vi "working controller not circlre.vi"() -> ()   [LabVIEW 2017]
uses:
  <vilib>/Simulation/Scripting/Companion Diagram/SimConfigNode/SimParams.ctl
  <vilib>/Simulation/Scripting/Companion Diagram/SimConfigNode/_simSolvers.ctl
  <vilib>/Simulation/Implementation/Shared/SIMSCR Execution Mode.ctl
  <vilib>/Simulation/Param Hierarchy/Typedefs/SIMPH Param Control Actions.ctl
  <vilib>/Simulation/Implementation/Shared/NILVSim_ParamChanged.vi
  <vilib>/Simulation/Implementation/Shared/NILVSIM_BeginStep.vi
  <vilib>/Simulation/Implementation/Shared/NILVSim_Manager.vi
  <vilib>/Utility/error.llb/Clear Errors.vi
  <vilib>/Simulation/Implementation/Shared/NILVSim_FinalizeModel.vi
  <vilib>/DAQmx/read.llb/DAQmx Read (Counter DBL 1Chan 1Samp).vi
  <vilib>/DAQmx/read.llb/DAQmx Read (Digital Bool 1Line 1Point).vi
  917b7e52-755f-4d44-bea8-9e7c9beac24e.vi
  a58f9967-76f1-4ebc-ad3d-26e75a3ca160.vi
  <vilib>/DAQmx/write.llb/DAQmx Write (Analog DBL 1Chan 1Samp).vi
  <vilib>/DAQmx/create/channels.llb/DAQmx Create Channel (AO-Voltage-Basic).vi
  <vilib>/DAQmx/create/channels.llb/DAQmx Create Channel (DI-Digital Input).vi
  <vilib>/DAQmx/create/channels.llb/DAQmx Create Channel (CI-Count Edges).vi
  <vilib>/Simulation/Implementation/Shared/SIM Unbundle Sim Info.vi
  <vilib>/Simulation/Implementation/Shared/NILVSim_Initialize.vi
  <vilib>/Simulation/Utility/Implementation/NILVSim Get Time and IsAcceptedStep.vi
  <vilib>/Simulation/Implementation/Shared/SIMSH Read Queue.vi
  <vilib>/Simulation/Implementation/Shared/NILVSim_GetModelError.vi
  <vilib>/Simulation/Implementation/Shared/SIM Bundle Sim Info.vi
  <vilib>/DAQmx/miscellaneous.llb/DAQmx Fill In Error Info.vi
  <vilib>/Simulation/Implementation/XNodeFramework/SimXNode/SimX.xnode
  <vilib>/Simulation/Model Libraries/PID/SIM PID (Parallel).vi
  <vilib>/Simulation/Model Libraries/PID/SIM PID.vi
  <vilib>/Simulation/Scripting/Companion Diagram/SimConfigNode/SimDog.xnode
  <vilib>/Simulation/Model Libraries/PID/SIM PID (Academic).vi
  <vilib>/Simulation/Implementation/Shared/NI_SIM_Implementation.lvlib
panel:
  out "down":bool
  out "right":bool
  out "x entered":dbl
  out "y enetred":dbl
  out "Numeric 2":i32
  out "greater -1 x":bool
  out "less 1 x":bool
  out "d":bool
  out "c":bool
  out "b":bool
  out "direction selected":dbl
  out "circle reset":bool
  in  "part circle":T1(ring)=enum."a"
  in  "Raduis":dbl
  out "at 2f":bool
  out "Step 2J":bool
  out "Step 2H":bool
  out "Shape drawing steps":enum16{"corner", "1st switch", "reverse"}(ring)
  out "Step 2D":bool
  out "Step 2C":bool
  out "c":bool
  in  "height":dbl
  in  "length":dbl
  in  "part":T2(ring)=enum."a"
  out "Step 2A":bool
  out "Step 2B":bool
  in  "Has encoders been reset?":enum16{"don't reset", "reset"}(ring)
  out "x distance currently being travelled":dbl
  out "y distance currently being travelled":dbl
  out "error calced":dbl
  out "p1 dis 2":dbl
  out "p1 dis":dbl
  out "error y":dbl
  out "calc distance y":dbl
  out "calc distanc x":dbl
  out "error x":dbl
  out "reached y":bool
  out "reached x":bool
  out "Numeric":dbl
  in  "Draw rectangle":bool
  in  "Draw circle":bool
  out "In drawing mode":bool
  in  "Right-Down":bool
  in  "Left-Up":bool
  in  "Left-Down":bool
  in  "Right-Up":bool
  in  "right":bool
  in  "left":bool
  in  "motor 2":dbl(slide)=1.5 scale=-10.0..10.0
  in  "down":bool
  in  "up":bool
  in  "Y Length":dbl=30.0
  in  "X Length":dbl=30.0
  in  "Motor 2 encoder":tag="Dev1/ctr1"
  out "Pulses M2":dbl format="%.2f"
  in  "Motor 1 encoder":tag="Dev1/ctr0"
  out "Pulses M1":dbl format="%.2f"
  out "Right":bool
  out "Bottom":bool
  out "Left":bool
  out "Top":bool
  in  "Switch 4/Line 3":tag="Dev1/port0/line3"
  in  "Switch 3/Line 2":tag="Dev1/port0/line2"
  in  "Switch 2/Line 1":tag="Dev1/port0/line1"
  in  "Switch 1/Line 0":tag="Dev1/port0/line0"
  in  "Motor stop":bool
  in  "Motor 1":tag="Dev1/ao0"
  in  "max Voltage":dbl=10.0
  in  "Min Voltage":dbl=-10.0
  in  "Motor 2":tag="Dev1/ao1"
  in  "motor 1":dbl(slide)=1.5 scale=-10.0..10.0
  in  "stop":bool
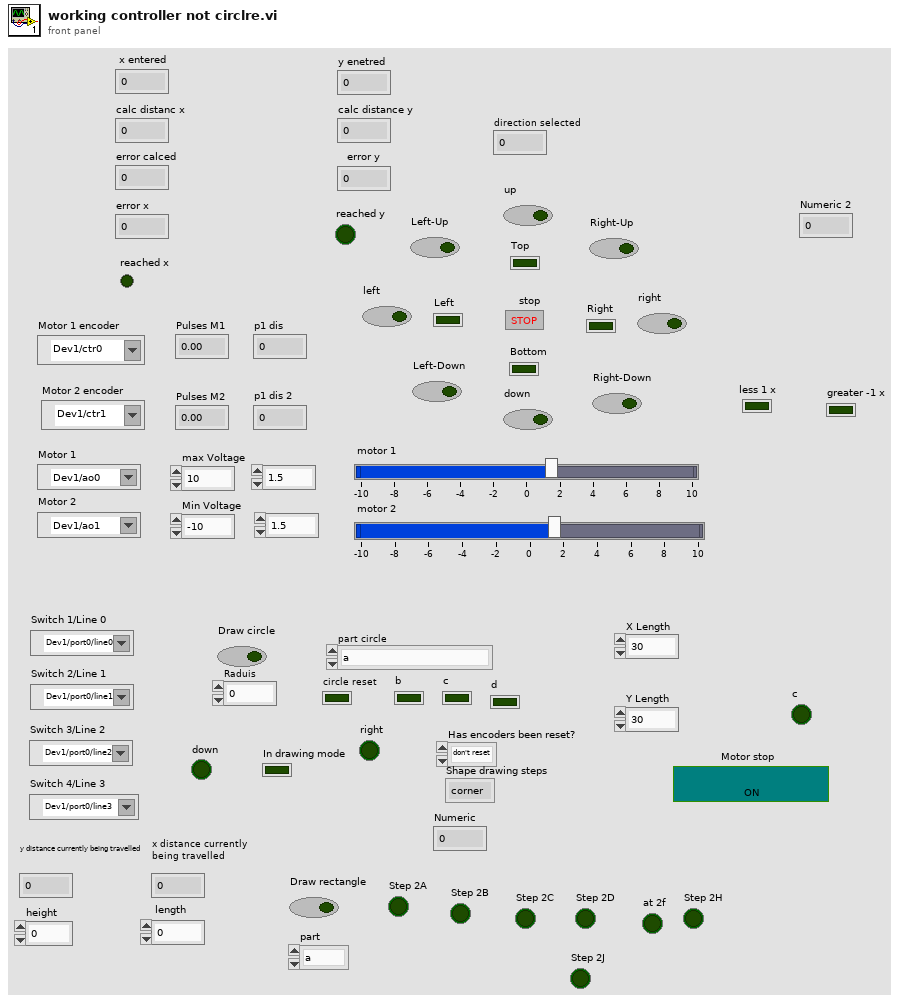
[diagram p1: front panel]
types:
  T1 = enum16{"d", "c", "b", "going right", "going down", "a"}
  T2 = enum16{"nothing", "j", "i", "h", "g", "f", "e", "d", "c", "b", "a"}
  T3 = enum16{"Simulate to Completion", "Single Time-Step Simulation (Fixed Step Only)"}
  T4 = typedef "SIMSCR Execution Mode.ctl" = enum16{"Simulate to Completion", "Single Time-Step Simulation (Fixed Step Only)"}
  T5 = typedef "SIMPH Param Control Actions.ctl" = enum16{"get params", "set params"}
  T6 = cluster{"SIMSH Sim Time":dbl, "SIM PID Derivative Gain.vi":cluster{"output":dbl}, "SIM PID Derivative Gain.vi - SIMSH":cluster{"SIMSH Sim Time":dbl, "t 3":dbl, "Select 2":cluster{"s? t:f":dbl}, "Equal?":cluster{"x = y?":bool}, "Or":cluster{"x .or. y?":bool}, "Equal To 0?":cluster{"x = 0?":bool}}, "High Frequency [s] (Tf)":dbl, "Gain":cluster{"output":dbl}, "Summation":cluster{"Result":dbl}, "Integral Gain - series.vi":cluster{"output":dbl}, "Integral Gain - series.vi - SIMSH":cluster{"SIMSH Sim Time":dbl, "Select 2":cluster{"s? t:f":dbl}, "integral in gain?":bool, "Integrator":cluster{"output y(t)":dbl}, "Gain 2":cluster{"output":dbl}, "Select":cluster{"s? t:f":dbl}, "Equal To 0?":cluster{"x = 0?":bool}, "Reciprocal":cluster{"1/x":dbl}}}
  T7 = typedef "SimParams.ctl" = cluster{"Initial Time (s)":dbl, "Final Time (s)":dbl, "Step Size (s)":dbl, "ODE Solver":T8, "Minimum Step Size (s)":dbl, "Maximum Step Size (s)":dbl, "Relative Tolerance":dbl, "Absolute Tolerance":dbl, "Software Timing":bool, "Initial Step Size (s)":dbl, "Automatic Fixed Step Size?":bool, "Automatic Discrete Step Size?":bool, "Discrete Step Size (s)":dbl, "Calculate using Time Step":bool, "Solver Wired?":bool, "Prev.Frm.Expected End":u64, "Prev.Frm.Actual End":u64, "Prev.Frm.Finished Late?":bool, "Prev.Iter.Expected End":u64, "Prev.Iter.Actual End":u64, "Prev.Iter.Finished Late?":bool, "Expected Iteration Start":u64, "Actual Iteration Start":u64, "Expected Frame Start":u64, "Actual Frame Start":u64, "Source Name":string, "Name":string, "Period":i64, "Deadline":i64, "Offset":i64, "Start":i64, "Priority":i32, "Timeout":i32, "Processor":i32, "Mode":enum32{"No Change", "Process missed periods, maintain original phase", "Discard missed periods, maintain original phase", "Process missed periods, ignore original phase", "Discard missed periods, ignore original phase"}, "Wakeup reason":enum32{"Normal", "Aborted", "Asynchronous wakeup", "Timing source error", "Timed loop error", "Timeout"}, "Error":errorcluster, "Source Type":string, "Secondary Source Type":string, "Global End Time":u64, "Global Start Time":u64, "Full Solver Reset":bool, "Execution Mode":T4, "Nan/Inf Check":bool, "Custom Solver Library":string, "Solver Is Variable":bool, "custom solver name":string, "Signal Collection Decimation":u32}
  T8 = typedef "_simSolvers.ctl" = enum16{"Runge-Kutta 1 (Euler)", "Runge-Kutta 2", "Runge-Kutta 3", "Runge-Kutta 4", "Runge-Kutta 23 (variable)", "Runge-Kutta 45 (variable)", "BDF (variable)", "Adams-Moulton (variable)", "Rosenbrock (variable)", "Discrete States Only", "SDIRK 4 (variable)", "Radau 5 (variable)", "Radau 9 (variable)", "Radau 13 (variable)", "Radau [Variable Order] (variable)", "Gear's Method (variable)", "Linearizer", "State Query", "Trim Eval", "Custom Solver"}
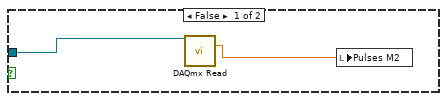
[diagram p2: hidden frame]
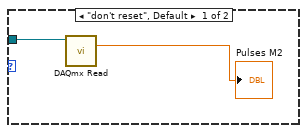
[diagram p3: hidden frame]
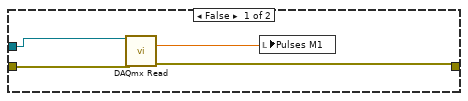
[diagram p4: hidden frame]
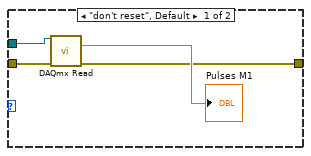
[diagram p5: hidden frame]
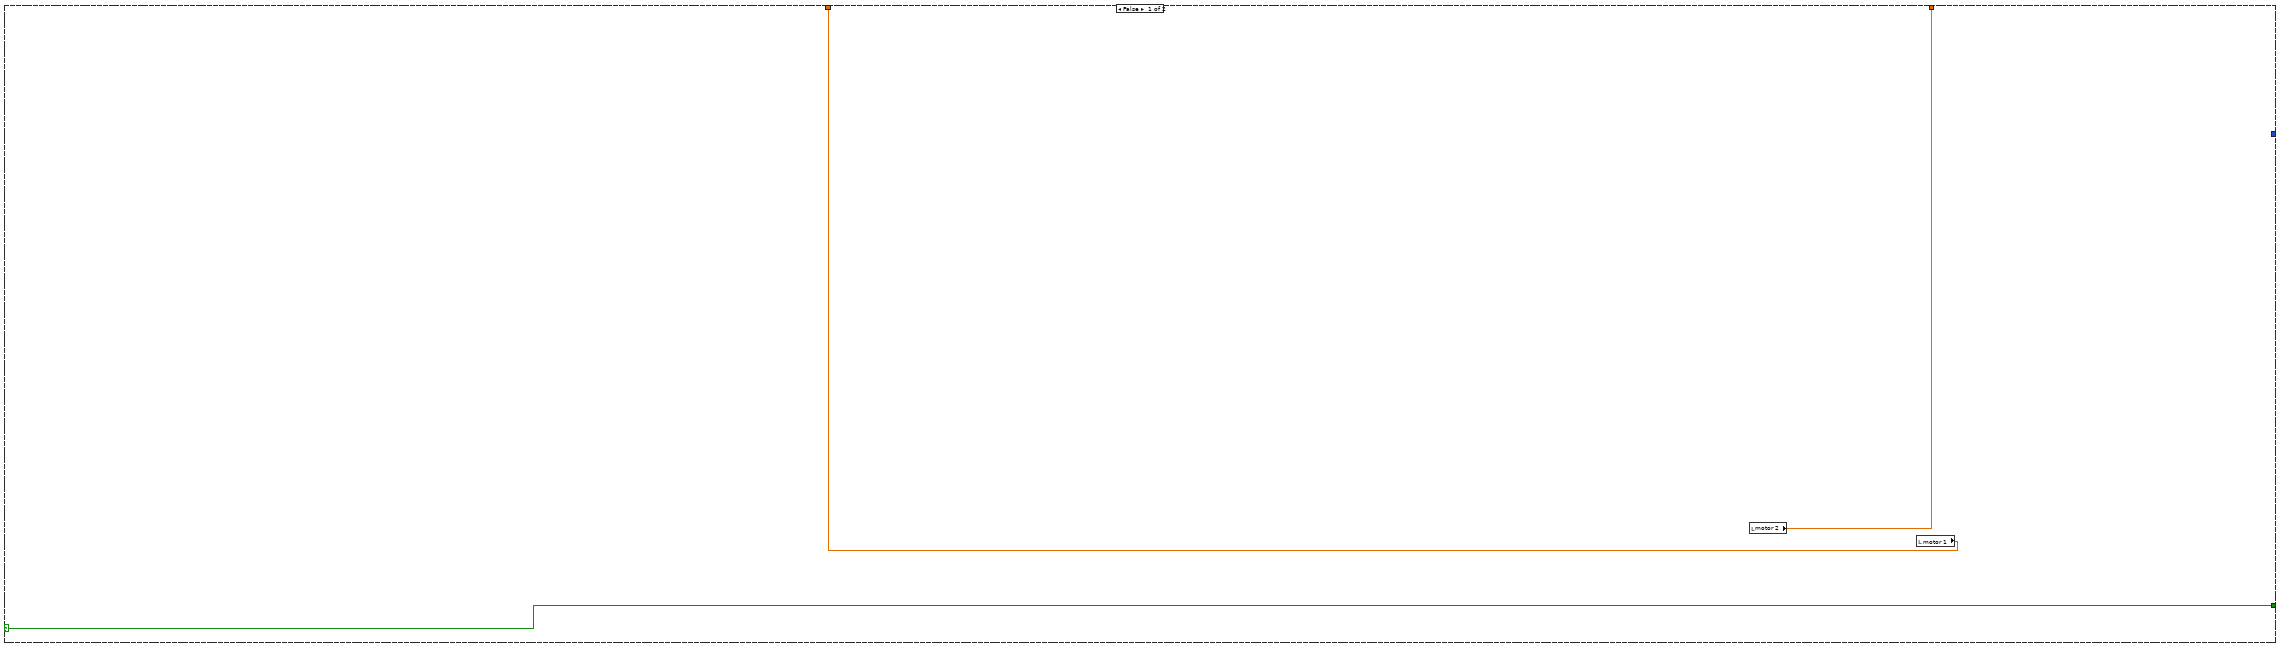
[diagram p6: hidden frame]
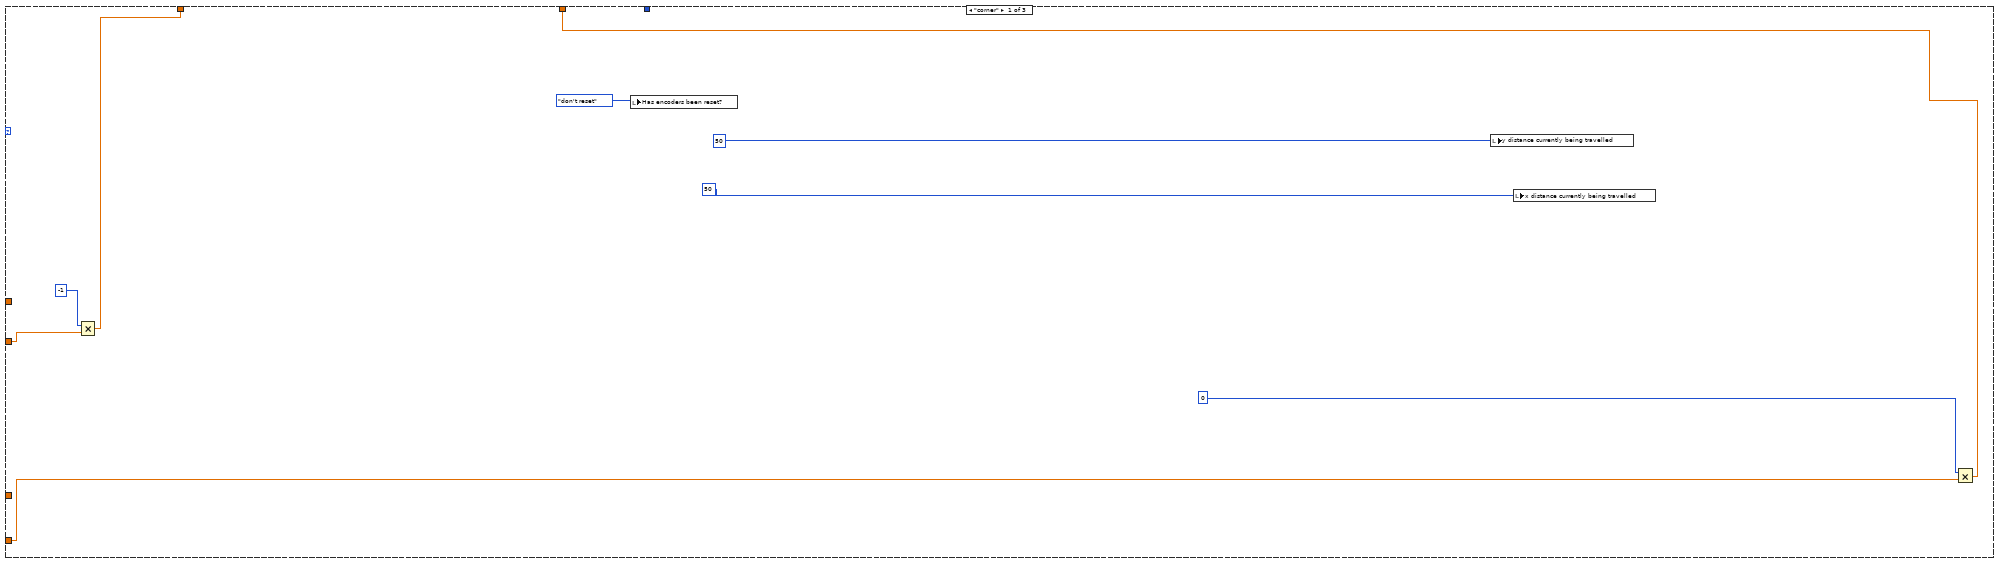
[diagram p7: hidden frame]
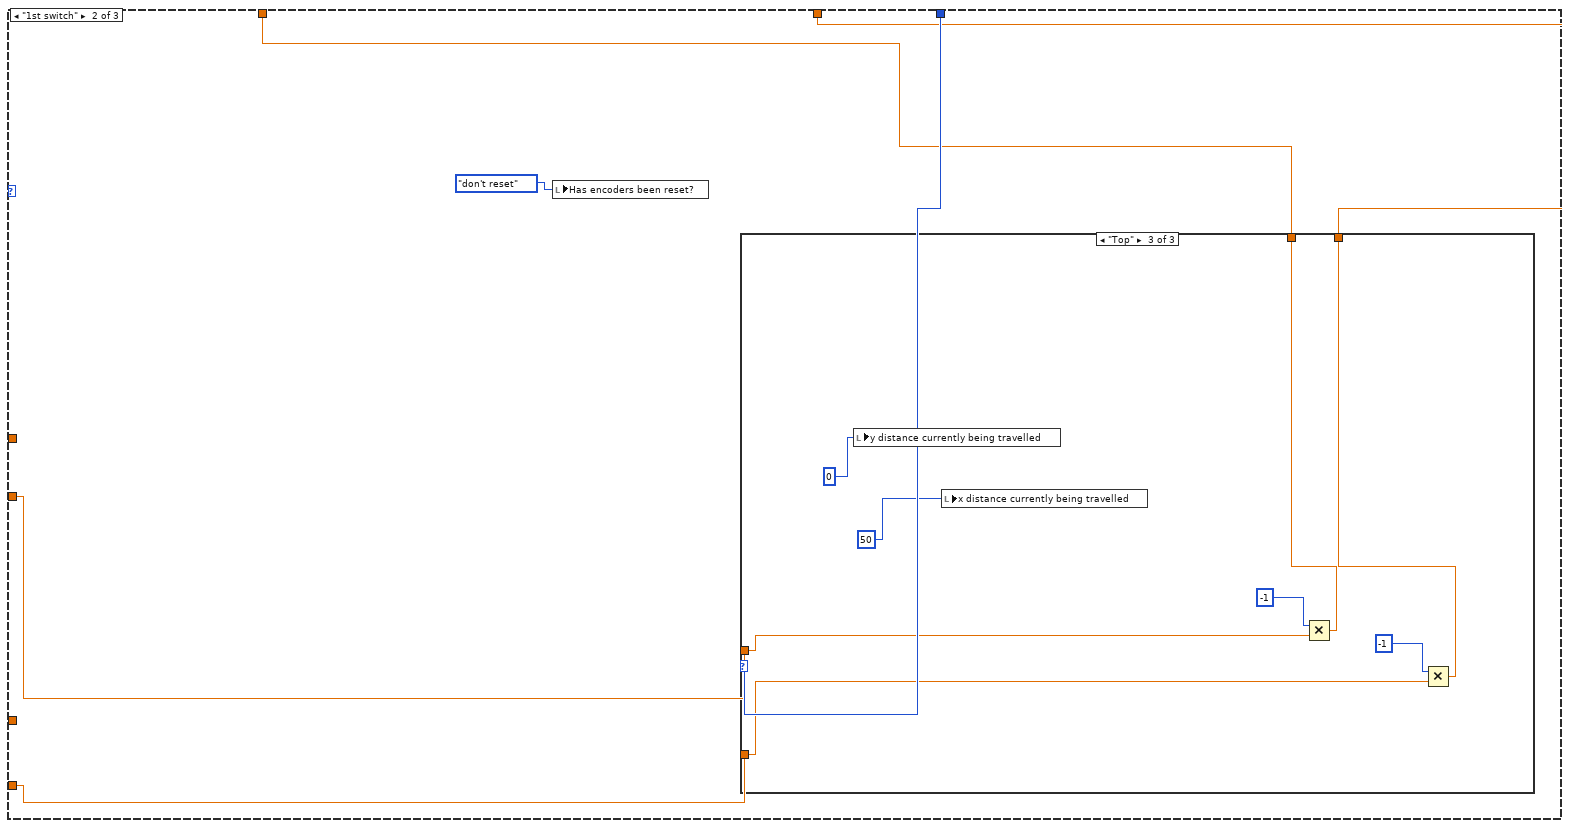
[diagram p8: hidden frame]
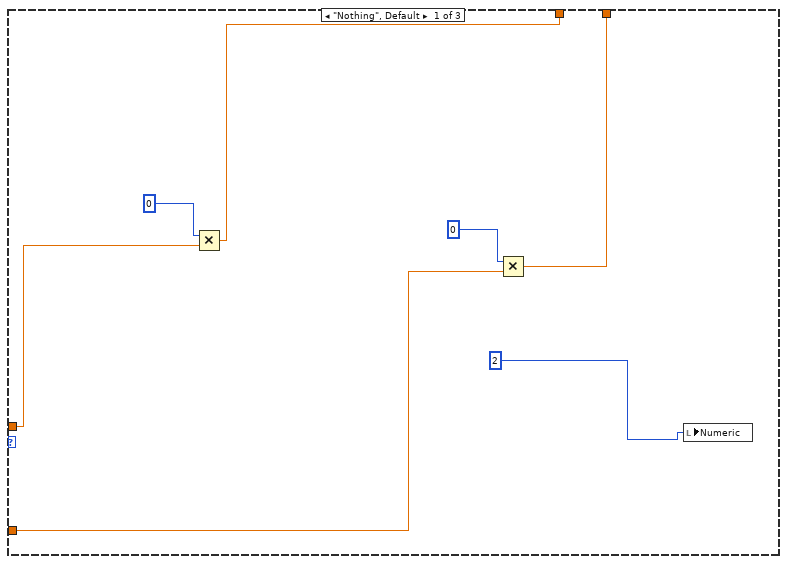
[diagram p9: hidden frame]
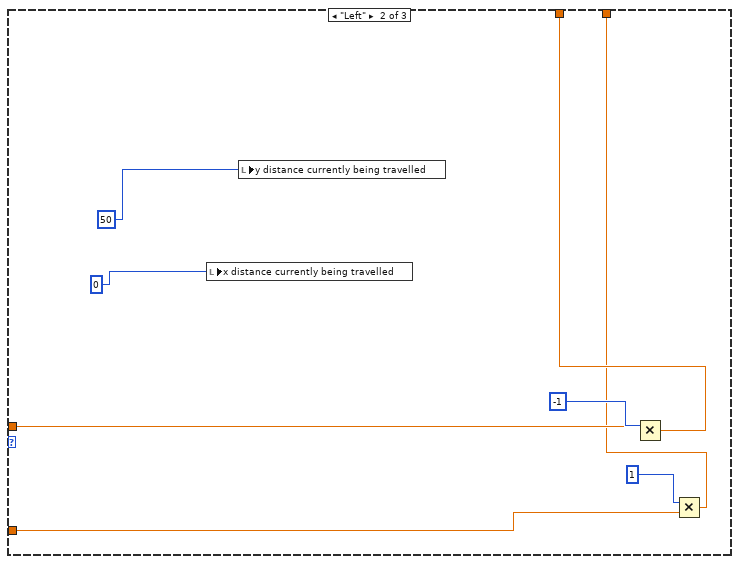
[diagram p10: hidden frame]
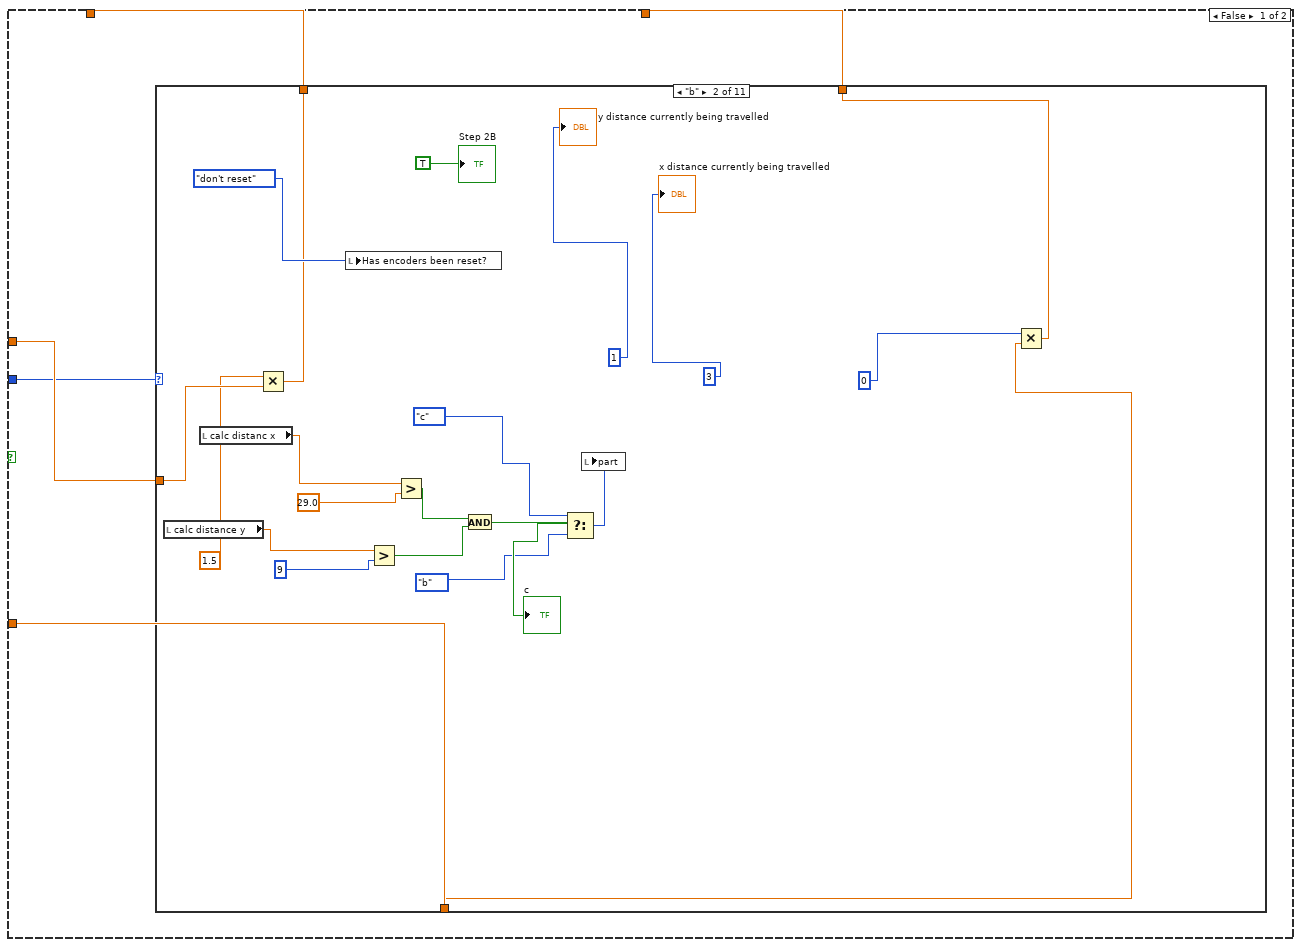
[diagram p11: hidden frame]
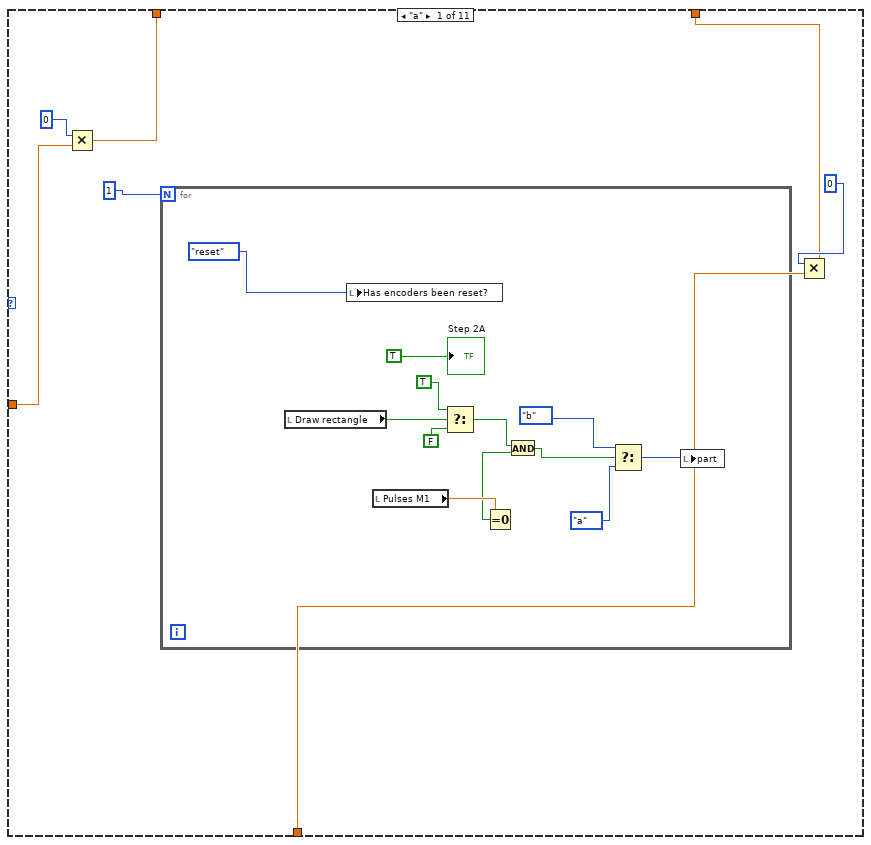
[diagram p12: hidden frame]
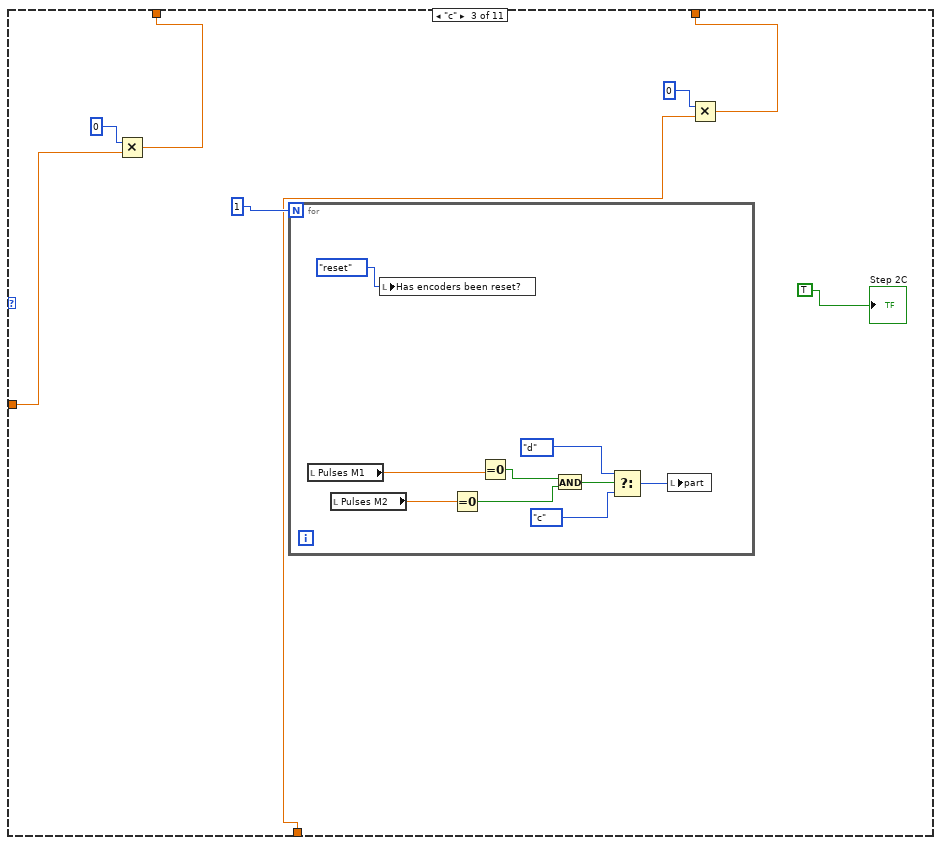
[diagram p13: hidden frame]
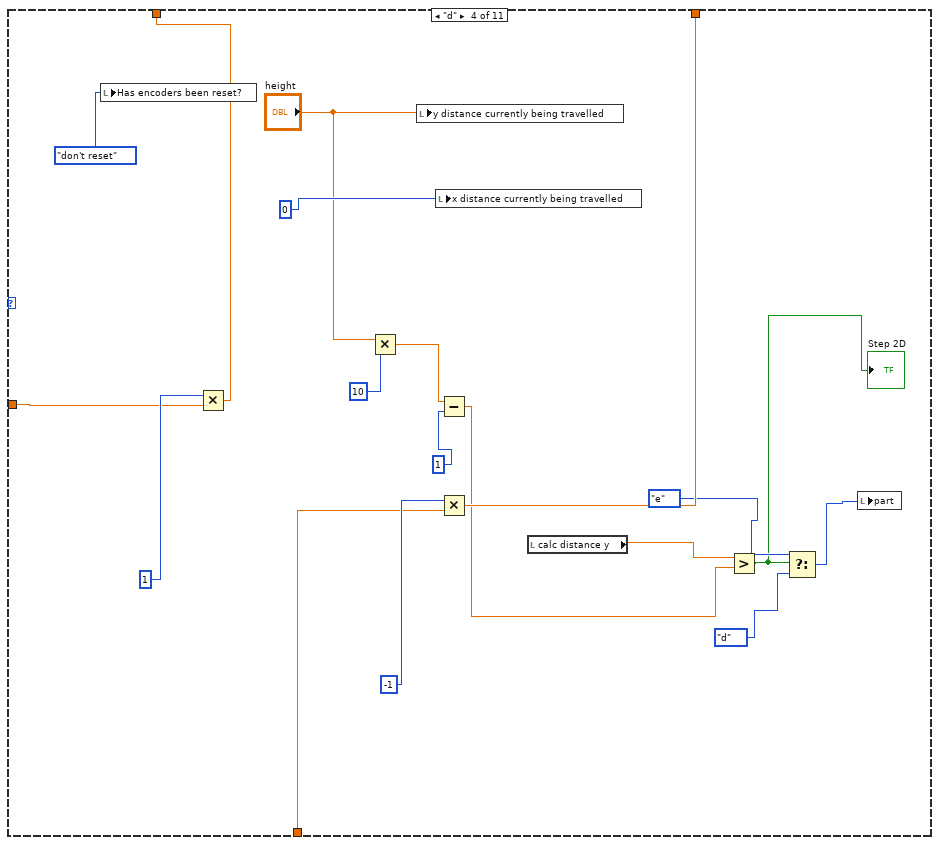
[diagram p14: hidden frame]
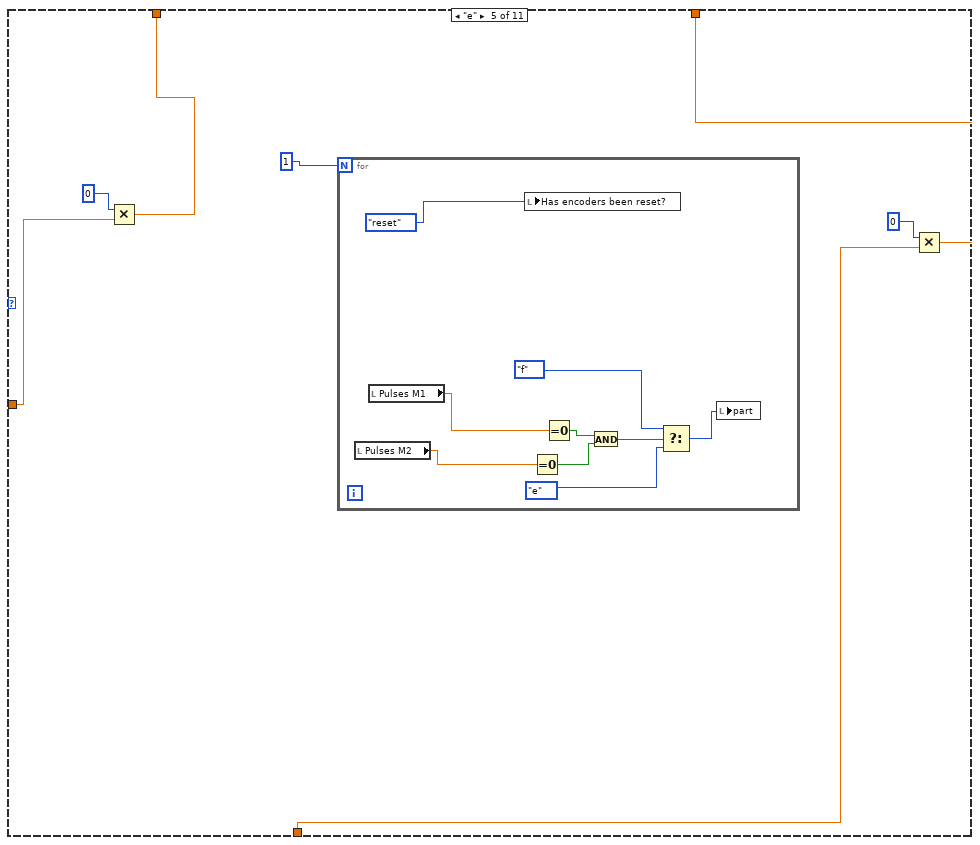
[diagram p15: hidden frame]
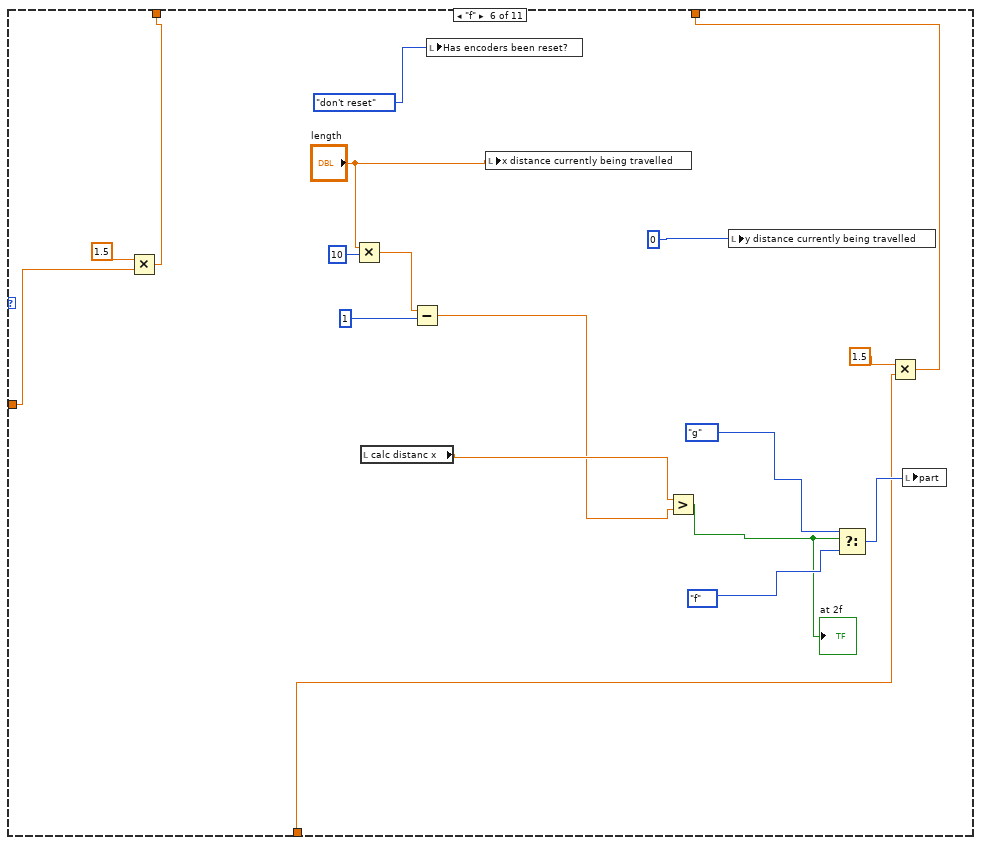
[diagram p16: hidden frame]
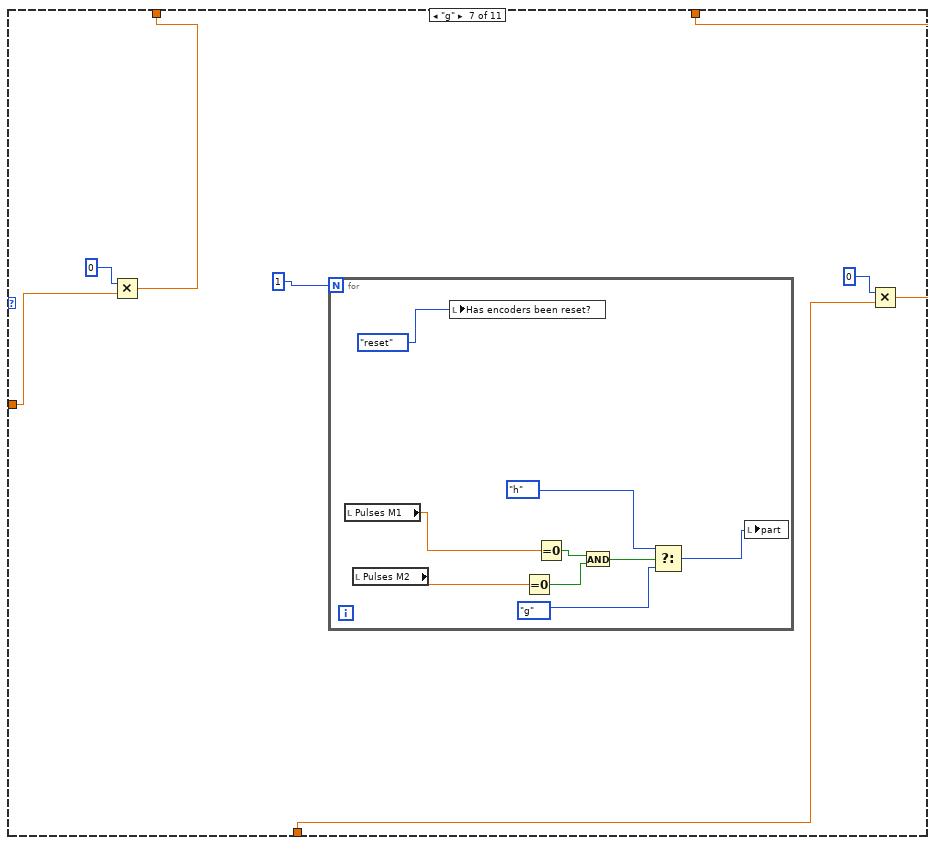
[diagram p17: hidden frame]
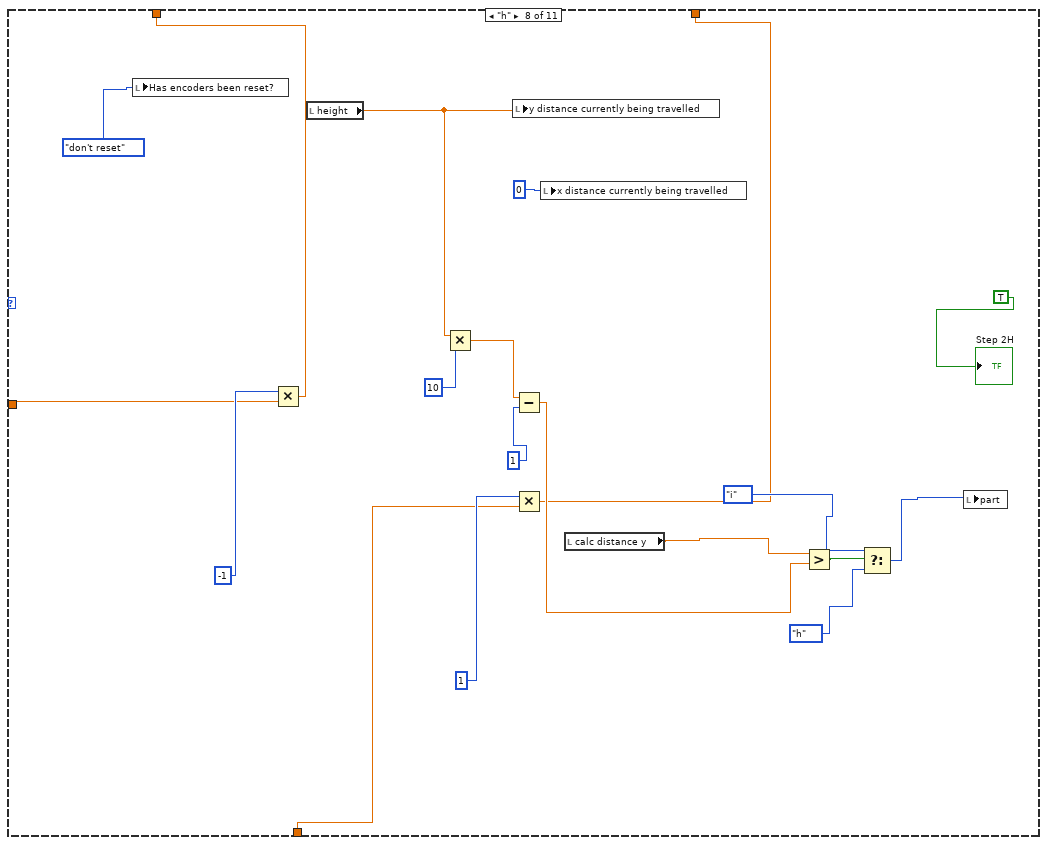
[diagram p18: hidden frame]
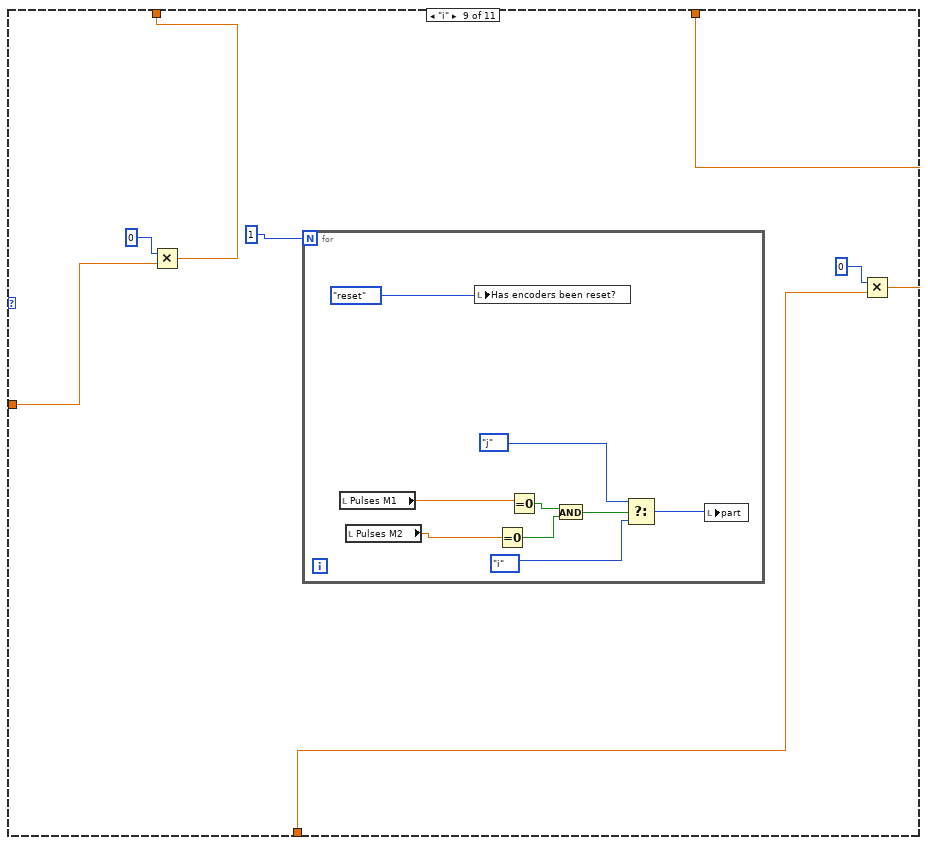
[diagram p19: hidden frame]
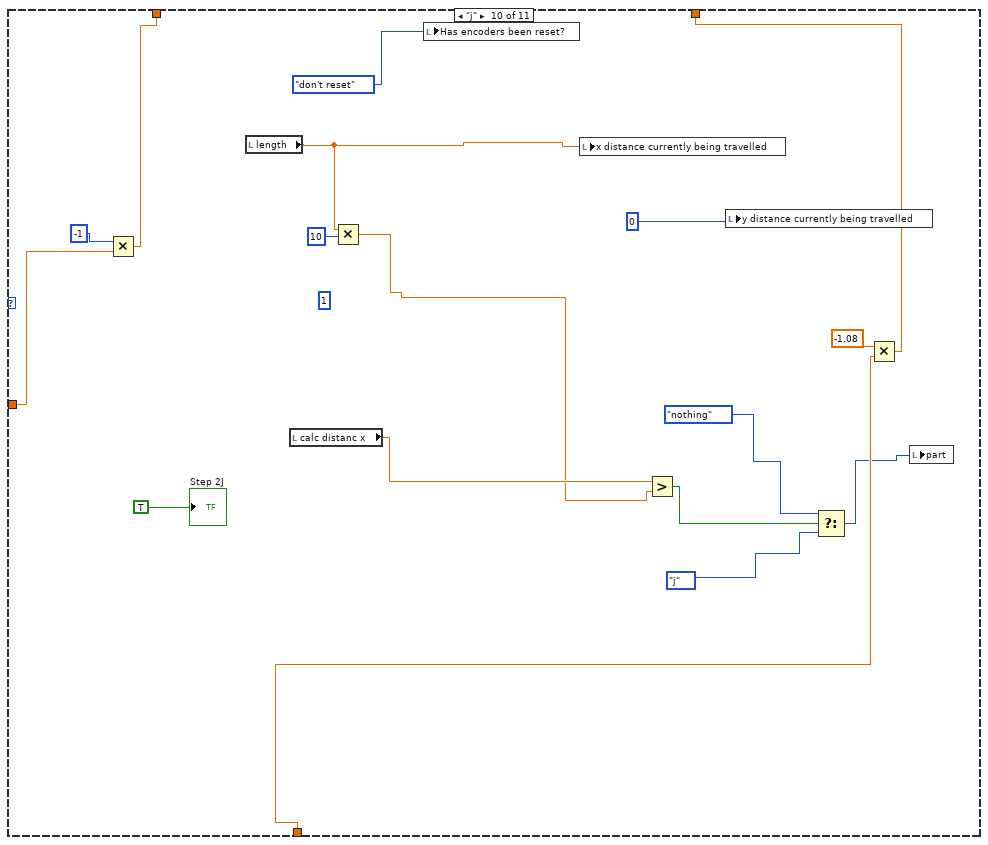
[diagram p20: hidden frame]
diagram:
  n1 = call-poly <vilib>:"DAQmx Create Virtual Channel.vi"("lines"="Switch 1/Line 0") -> ("task out"=w36:refnum<k21>, "error out"=w32:errorcluster)  [unwired: 13 in]
  n2 = call-poly <vilib>:"DAQmx Create Virtual Channel.vi"("lines"="Switch 2/Line 1") -> ("task out"=w35:refnum<k21>, "error out"=w31:errorcluster)  [unwired: 13 in]
  n3 = call-poly <vilib>:"DAQmx Create Virtual Channel.vi"("lines"="Switch 3/Line 2") -> ("task out"=w34:refnum<k21>, "error out"=w30:errorcluster)  [unwired: 13 in]
  n4 = call-poly <vilib>:"DAQmx Create Virtual Channel.vi"("lines"="Switch 4/Line 3") -> ("task out"=w33:refnum<k21>, "error out"=w29:errorcluster)  [unwired: 13 in]
  n5 = call <vilib>:"DAQmx Start Task.vi"("task/channels in"=w36, "error in"=w32) -> ("task out"=w28:refnum<k21>, "error out"=w26:errorcluster)  [unwired: 12 in]
  n6 = call <vilib>:"DAQmx Start Task.vi"("task/channels in"=w35, "error in"=w31) -> ("task out"=w24:refnum<k21>, "error out"=w21:errorcluster)  [unwired: 12 in]
  n7 = call <vilib>:"DAQmx Start Task.vi"("task/channels in"=w34, "error in"=w30) -> ("task out"=w23:refnum<k21>, "error out"=w20:errorcluster)  [unwired: 12 in]
  n8 = call <vilib>:"DAQmx Start Task.vi"("task/channels in"=w33, "error in"=w29) -> ("task out"=w22:refnum<k21>, "error out"=w19:errorcluster)  [unwired: 12 in]
  n9 = call-poly <vilib>:"DAQmx Create Virtual Channel.vi"("maximum value"="max Voltage", "minimum value"="Min Voltage", "physical channels"="Motor 1") -> ("task out"=w46:refnum<k21>, "error out"=w42:errorcluster)  [unwired: 11 in]
  n10 = call-poly <vilib>:"DAQmx Create Virtual Channel.vi"("counter"="Motor 2 encoder") -> ("task out"=w6:refnum<k21>)  [unwired: 13 in, 1 out]
  n11 = call-poly <vilib>:"DAQmx Create Virtual Channel.vi"("maximum value"="max Voltage", "minimum value"="Min Voltage", "physical channels"="Motor 2") -> ("task out"=w49:refnum<k21>, "error out"=w41:errorcluster)  [unwired: 11 in]
  n12 = call-poly <vilib>:"DAQmx Create Virtual Channel.vi"("counter"="Motor 1 encoder") -> ("task out"=w7:refnum<k21>, "error out"=w2:errorcluster)  [unwired: 13 in]
  n13 = call <vilib>:"DAQmx Start Task.vi"("task/channels in"=w6) -> ("task out"=w1:refnum<k21>)  [unwired: 13 in, 1 out]
  n14 = call <vilib>:"DAQmx Start Task.vi"("task/channels in"=w7) -> ("task out"=w3:refnum<k21>)  [unwired: 13 in, 1 out]
  n15 = while {
    tunnel: w49 -> [w243]
    tunnel: [w240] -> w48
    tunnel: w46 -> [w237]
    tunnel: [w236] -> w45
    tunnel: w42 -> [w234]
    tunnel: w41 -> [w233]
    tunnel: w28 -> [w227]
    tunnel: [w226] -> w27
    tunnel: w26 -> [w225]
    tunnel: [w224] -> w25
    tunnel: w24 -> [w223]
    tunnel: w23 -> [w222]
    tunnel: w22 -> [w221]
    tunnel: w21 -> [w220]
    tunnel: w20 -> [w219]
    tunnel: w19 -> [w218]
    tunnel: [w217] -> w18
    tunnel: [w216] -> w17
    tunnel: [w215] -> w16
    tunnel: [w214] -> w15
    tunnel: [w213] -> w14
    tunnel: [w212] -> w13
    tunnel: [w129] -> w10
    tunnel: w3 -> [w131]
    tunnel: w2 -> [w130]
    tunnel: w1 -> [w127]
    stop <- "stop" stop-if-true
    n16 = Or(x="Draw circle", y="Draw rectangle") -> (x .or. y?=w150:bool)
    n17 = local read "error y"() -> (w97:dbl)
    n18 = local read "error y"() -> (w96:dbl)
    n19 = local read "error x"() -> (w98:dbl)
    n20 = local read "error y"() -> (w112:dbl)
    n21 = local read "error y"() -> (w109:dbl)
    n22 = local read "error x"() -> (w105:dbl)
    n23 = local read "error x"() -> (w104:dbl)
    n24 = local read "error y"() -> (w113:dbl)
    n25 = local read "error x"() -> (w114:dbl)
    n26 = Less Than 0?(x=w97) -> (x < 0?=w95:bool)
    n27 = Less Than 0?(x=w98) -> (x < 0?=w94:bool)
    n28 = Greater Than 0?(x=w96) -> (x > 0?=w93:bool)
    n29 = Less Than 0?(x=w109) -> (x < 0?=w107:bool)
    n30 = Equal To 0?(x=w114) -> (x = 0?=w108:bool)
    n31 = Greater Than 0?(x=w112) -> (x > 0?=w111:bool)
    n32 = local read "error y"() -> (w90:dbl)
    n33 = local read "error x"() -> (w89:dbl)
    n34 = Greater Than 0?(x=w105) -> (x > 0?=w103:bool)
    n35 = Equal To 0?(x=w113) -> (x = 0?=w102:bool)
    n36 = Less Than 0?(x=w104) -> (x < 0?=w101:bool)
    n37 = And(x=w95, y=w94) -> (x .and. y?=w91:bool)
    n38 = And(x=w94, y=w93) -> (x .and. y?=w92:bool)
    n39 = And(x=w111, y=w108) -> (x .and. y?=w110:bool)
    n40 = And(x=w108, y=w107) -> (x .and. y?=w106:bool)
    n41 = local read "error y"() -> (w85:dbl)
    n42 = And(x=w103, y=w102) -> (x .and. y?=w100:bool)
    n43 = And(x=w102, y=w101) -> (x .and. y?=w99:bool)
    n44 = Greater Than 0?(x=w90) -> (x > 0?=w88:bool)
    n45 = Greater Than 0?(x=w89) -> (x > 0?=w86:bool)
    n46 = Less Than 0?(x=w85) -> (x < 0?=w84:bool)
    n47 = And(x=w88, y=w86) -> (x .and. y?=w87:bool)
    n48 = And(x=w86, y=w84) -> (x .and. y?=w83:bool)
    n49 = Select(t=1, s=w110, f=0) -> (s? t:f=w196:i32)
    n50 = Select(t=10, s=w99, f=0) -> (s? t:f=w194:i32)
    n51 = Select(t=2, s=w106, f=0) -> (s? t:f=w195:i32)
    n52 = Select(t=100, s=w87, f=0) -> (s? t:f=w192:i32)
    n53 = Select(t=200, s=w91, f=0) -> (s? t:f=w191:i32)
    n54 = Select(t=20, s=w100, f=0) -> (s? t:f=w193:i32)
    n55 = Select(t=1000, s=w92, f=0) -> (s? t:f=w190:i32)
    n56 = Select(t=2000, s=w83, f=0) -> (s? t:f=w176:i32)
    n57 = Add(x=w196, y=w195) -> (x+y=w189:i32)
    n58 = Add(x=w194, y=w193) -> (x+y=w188:i32)
    n59 = Add(x=w192, y=w191) -> (x+y=w187:i32)
    n60 = Add(x=w190, y=w176) -> (x+y=w175:i32)
    n61 = Add(x=w189, y=w188) -> (x+y=w186:i32)
    n62 = local read "y distance currently being travelled"() -> (w133:dbl)
    n63 = Add(x=w187, y=w175) -> (x+y=w174:i32)
    n64 = local read "Draw rectangle"() -> (w141:bool)
    n65 = local read "Draw circle"() -> (w142:bool)
    n66 = call-poly <vilib>:"DAQmx Read.vi"("task/channels in"=w227, "error in"=w225) -> ("task out"=w226:refnum<k21>, "data"=w152:bool, "error out"=w224:errorcluster)  [unwired: 11 in]
    "Top" <- w152
    n67 = call-poly <vilib>:"DAQmx Read.vi"("task/channels in"=w223, "error in"=w220) -> ("task out"=w217:refnum<k21>, "data"=w161:bool, "error out"=w214:errorcluster)  [unwired: 11 in]
    "Bottom" <- w161
    n68 = call-poly <vilib>:"DAQmx Read.vi"("task/channels in"=w222, "error in"=w219) -> ("task out"=w216:refnum<k21>, "data"=w160:bool, "error out"=w213:errorcluster)  [unwired: 11 in]
    "Right" <- w160
    n69 = call-poly <vilib>:"DAQmx Read.vi"("task/channels in"=w221, "error in"=w218) -> ("task out"=w215:refnum<k21>, "data"=w159:bool, "error out"=w212:errorcluster)  [unwired: 11 in]
    "Left" <- w159
    n70 = Add(x=w186, y=w174) -> (x+y=w82:i32)
    "direction selected" <- w82
    n71 = Or(x=w142, y=w141) -> (x .or. y?=w140:bool)
    n72 = Select(t=w133, s=w140, f="Y Length") -> (s? t:f=w138:dbl)
    n73 = Multiply(x=w138, y=10) -> (x*y=w52:dbl)
    "y enetred" <- w52
    n74 = local read "Pulses M1"() -> (w128:dbl)
    n75 = local read "Pulses M2"() -> (w143:dbl)
    n76 = Divide(x=w128, y=52.56) -> (x/y=→"p1 dis":dbl)
    n77 = feedback #1() -> (w56:dbl)  [unwired: 1 in]
    "calc distance y" <- w56
    n78 = formula code="if (Ylength==0)\nYerror=0;\n else  \nif(Ylength<0)\nYerror= Ylength+calculating_y_dis;\nelse\nYerror= Ylength-calculating_y_dis;\n\nif (calculating_y_dis>1000)\nstay=0;\nif (stay==0 )\nYerror=0;"("Ylength"=w52, "calculating_y_dis"=w56, "stay"=1) -> ("Yerror"=w116:dbl)
    n79 = Divide(x=w143, y=52.56) -> (x/y=→"p1 dis 2":dbl)
    n80 = formula code="X=((PulseM1/52.56)+(PulseM2/52.56))/2.0;\nY=((PulseM1/52.56)+(PulseM2/52.56))/2.0;"("PulseM1"=w128, "PulseM2"=w143) -> ("X"=w61:dbl, "Y"=w65:dbl)
    n81 = local read "x distance currently being travelled"() -> (w132:dbl)
    n82 = local read "Draw rectangle"() -> (w135:bool)
    n83 = Multiply(x=1000, y=w65) -> (x*y=w68:dbl)
    n84 = local read "Draw circle"() -> (w134:bool)
    n85 = xnode "PID"("Error"=w116) -> ("Output"=w67:dbl)  [unwired: 2 in, 11 out]
    n86 = Or(x=w135, y=w134) -> (x .or. y?=w123:bool)
    n87 = Select(t=w132, s=w123, f="X Length") -> (s? t:f=w136:dbl)
    n88 = Multiply(x=w136, y=10) -> (x*y=w51:dbl)
    "x entered" <- w51
    n89 = Multiply(x=1000, y=w61) -> (x*y=w62:dbl)
    n90 = Greater?(x=1, y=w67) -> (0:w80:bool)
    n91 = Less?(x=-1, y=w67) -> (x < y?=w78:bool)
    n92 = case shown="0, Default" w82 {
      tunnel: "motor 1" -> [w1094 w1097 w1100 w1107 w1111 w1115 w1121 w1127 w1133 w1138 w1145]
      tunnel: "motor 2" -> [w1091 w1099 w1102 w1105 w1110 w1113 w1119 w1125 w1131 w1139 w1144]
      tunnel: [w1090 w1099 w1101 w1104 w1110 w1112 w1118 w1124 w1130 w1136 w1143] -> w168
      tunnel: [w1093 w1096 w1100 w1106 w1111 w1114 w1120 w1126 w1132 w1137 w1142] -> w170
      frame 0, Default {
        n93 = Multiply(x=0, y=w1094) -> (x*y=w1093:dbl)
        n94 = Multiply(x=0, y=w1091) -> (x*y=w1090:dbl)
      }
      frame 1 {
        n95 = Multiply(x=-1, y=w1097) -> (x*y=w1096:dbl)
      }
      frame 2 {
        n96 = Multiply(x=-1.003, y=w1102) -> (x*y=w1101:dbl)
      }
      frame 10 {
        n97 = Multiply(x=-1, y=w1107) -> (x*y=w1106:dbl)
        n98 = Multiply(x=-1.1, y=w1105) -> (x*y=w1104:dbl)
      }
      frame 20 {
      }
      frame 100 {
        n99 = Multiply(x=0, y=w1115) -> (x*y=w1114:dbl)
        n100 = Multiply(x=1, y=w1113) -> (x*y=w1112:dbl)
      }
      frame 200 {
        n101 = Multiply(x=0, y=w1121) -> (x*y=w1120:dbl)
        n102 = Multiply(x=-1, y=w1119) -> (x*y=w1118:dbl)
      }
      frame 1000 {
        n103 = Multiply(x=-1, y=w1127) -> (x*y=w1126:dbl)
        n104 = Multiply(x=0, y=w1125) -> (x*y=w1124:dbl)
      }
      frame 2000 {
        n105 = Multiply(x=1, y=w1133) -> (x*y=w1132:dbl)
        n106 = Multiply(x=0, y=w1131) -> (x*y=w1130:dbl)
      }
      frame 4000 {
        n107 = Multiply(x=-1, y=w1138) -> (x*y=w1137:dbl)
        n108 = Multiply(x=0, y=w1139) -> (x*y=w1136:dbl)
      }
      frame 8000 {
        n109 = Multiply(x=-1, y=w1145) -> (x*y=w1142:dbl)
        n110 = Multiply(x=0, y=w1144) -> (x*y=w1143:dbl)
      }
    }
    n111 = And(x=w80, y=w78) -> (x .and. y?=w66:bool)
    "reached y" <- w66
    n112 = Select(t=w68, s=w66, f=w65) -> (s? t:f=w64:dbl)
    n113 = feedback-in #1(w64) -> ()
    n114 = Multiply(x=0, y=w67) -> (x*y=w76:dbl)
    n115 = Select(t=w76, s=w66, f=w67) -> (s? t:f=→"error y":dbl)
    n116 = local read "Numeric"() -> (w120:dbl)
    n117 = Or(x=w161, y=w160) -> (x .or. y?=w210:bool)
    n118 = local read "Draw circle"() -> (w125:bool)
    n119 = local read "Draw rectangle"() -> (w124:bool)
    n120 = And(x=w159, y=w152) -> (x .and. y?=w121:bool)
    n121 = Exclusive Or(1:w152, 2:w159) -> (0:w166:bool)
    n122 = Select(t=1, s=w159, f=0) -> (s? t:f=w151:i32)
    n123 = Select(t=2, s=w152, f=w151) -> (s? t:f=w156:i32)
    n124 = Select(t=1, s=w166, f=w120) -> (s? t:f=w165:dbl)
    n125 = Select(t=2, s=w121, f=w165) -> (s? t:f=w163:dbl)
    n126 = feedback #2() -> (w59:bool)  [unwired: 1 in]
    "reached x" <- w59
    n127 = Select(t=w62, s=w59, f=w61) -> (s? t:f=w55:dbl)
    "calc distanc x" <- w55
    n128 = formula code="if (desired_xlength==0)\nXerror=0;\nelse\nif(desired_xlength>0)\nXerror=desired_xlength-actual_xLength;\nelse\nXerror=desired_xlength+actual_xLength;\n\nif (actual_xLength>1000)\nstay1=0;\nif (stay1==0)\nXerror=0;"("actual_xLength"=w55, "desired_xlength"=w51, "stay1"=1) -> ("Xerror"=w115:dbl)
    "error calced" <- w115
    n129 = xnode "PID 2"("Error"=w115) -> ("Output"=w71:dbl)  [unwired: 2 in, 11 out]
    n130 = Greater?(x=1, y=w71) -> (0:w57:bool)
    "greater -1 x" <- w57
    n131 = Less?(x=-1, y=w71) -> (x < y?=w58:bool)
    "less 1 x" <- w58
    n132 = And(x=w57, y=w58) -> (x .and. y?=w60:bool)
    n133 = Multiply(x=0, y=w71) -> (x*y=w73:dbl)
    n134 = feedback-in #2(w60) -> ()
    n135 = Or(x=w125, y=w124) -> (x .or. y?=w126:bool)
    n136 = Select(t=w73, s=w59, f=w71) -> (s? t:f=→"error x":dbl)
    n137 = call "Number To Enum.vim"("number"=w156, "enum type"=enum16{"Nothing", "Left", "Top"}."Nothing") -> ("number as enum"=w153:enum16{"Nothing", "Left", "Top"})
    n138 = case shown="True" w150 {
      selector: w150 -> [w770 w778]
      tunnel: [w770 w778] -> w173
      tunnel: [w769 w780] -> w172
      tunnel: [w768 w779] -> w171
      tunnel: w153 -> [_ w771]
      frame False {
        n139 = local read "motor 2"() -> (w768:dbl)
        n140 = local read "motor 1"() -> (w769:dbl)
      }
      frame True {
        n141 = local read "Numeric"() -> (w776:dbl)
        n142 = local read "Shape drawing steps"() -> (w773:enum16{"corner", "1st switch", "reverse"})
        n143 = Equal?(x=w776, y=2) -> (x = y?=w775:bool)
        n144 = Select(t=enum16{"corner", "1st switch", "reverse"}."reverse", s=w775, f=w773) -> (s? t:f=w772:enum16{"corner", "1st switch", "reverse"})
        n145 = local read "motor 2"() -> (w781:dbl)
        n146 = local read "motor 1"() -> (w782:dbl)
        n147 = case shown="\"reverse\"" w772 {
          tunnel: w771 -> [_ w797 _]
          tunnel: w782 -> [w789 w796 _]
          tunnel: w781 -> [w788 w795 _]
          tunnel: w782 -> [_ _ w827]
          tunnel: w781 -> [_ _ w826]
          tunnel: [w785 w794 w825] -> w780
          tunnel: [w784 w793 w824] -> w779
          frame "corner" {
            n148 = Multiply(x=-1, y=w789) -> (x*y=w785:dbl)
            n149 = local write "Has encoders been reset?"(enum16{"don't reset", "reset"}."don't reset") -> ()
            n150 = local write "y distance currently being travelled"(50) -> ()
            n151 = local write "x distance currently being travelled"(50) -> ()
            n152 = Multiply(x=0, y=w788) -> (x*y=w784:dbl)
          }
          frame "1st switch" {
            n153 = local write "Has encoders been reset?"(enum16{"don't reset", "reset"}."don't reset") -> ()
            n154 = case shown="\"Top\"" w797 {
              tunnel: [w802 w809 w818] -> w794
              tunnel: w796 -> [w804 w810 w816]
              tunnel: [w799 w807 w817] -> w793
              tunnel: w795 -> [w800 w808 w815]
              frame "Nothing", Default {
                n155 = Multiply(x=0, y=w804) -> (x*y=w802:dbl)
                n156 = Multiply(x=0, y=w800) -> (x*y=w799:dbl)
                n157 = local write "Numeric"(2) -> ()
              }
              frame "Left" {
                n158 = local write "x distance currently being travelled"(0) -> ()
                n159 = local write "y distance currently being travelled"(50) -> ()
                n160 = Multiply(x=-1, y=w810) -> (x*y=w809:dbl)
                n161 = Multiply(x=1, y=w808) -> (x*y=w807:dbl)
              }
              frame "Top" {
                n162 = local write "y distance currently being travelled"(0) -> ()
                n163 = local write "x distance currently being travelled"(50) -> ()
                n164 = Multiply(x=-1, y=w816) -> (x*y=w818:dbl)
                n165 = Multiply(x=-1, y=w815) -> (x*y=w817:dbl)
              }
            }
          }
          frame "reverse" {
            n166 = local read "Draw circle"() -> (w821:bool)
            n167 = case shown="True" w821 {
              tunnel: w827 -> [w832 w1017]
              tunnel: w826 -> [w831 w1016]
              tunnel: [w830 w1017] -> w825
              tunnel: [w829 w1016] -> w824
              tunnel: "part" -> [w828 _]
              frame False {
                n168 = case shown="\"b\"" w828 {
                  tunnel: w832 -> [w838 w868 w876 w904 w911 w928 w944 w965 w979 w1002 w1013]
                  tunnel: w831 -> [w835 w865 w874 w901 w907 w925 w941 w960 w976 w1000 w1011]
                  tunnel: [w836 w867 w875 w902 w910 w927 w945 w964 w980 w1001 w1012] -> w830
                  tunnel: [w833 w864 w873 w900 w908 w924 w942 w959 w977 w999 w1009] -> w829
                  frame "a" {
                    n169 = Multiply(x=0, y=w838) -> (x*y=w836:dbl)
                    n170 = for {
                      N: 1 -> [_]
                      n171 = local read "Draw rectangle"() -> (w840:bool)
                      n172 = local write "Has encoders been reset?"(enum16{"don't reset", "reset"}."reset") -> ()
                      n173 = local read "Pulses M1"() -> (w849:dbl)
                      n174 = Select(t=TRUE, s=w840, f=FALSE) -> (s? t:f=w843:bool)
                      n175 = Equal To 0?(x=w849) -> (x = 0?=w842:bool)
                      n176 = And(x=w843, y=w842) -> (x .and. y?=w841:bool)
                      n177 = Select(t=T2."b", s=w841, f=T2."a") -> (s? t:f=w848:T2)
                      n178 = local write "part"(w848) -> ()
                      "Step 2A" <- TRUE
                    }
                    n179 = Multiply(x=0, y=w835) -> (x*y=w833:dbl)
                  }
                  frame "b" {
                    n180 = local read "calc distance y"() -> (w852:dbl)
                    n181 = local read "calc distanc x"() -> (w853:dbl)
                    n182 = Multiply(x=1.5, y=w868) -> (x*y=w867:dbl)
                    n183 = local write "Has encoders been reset?"(enum16{"don't reset", "reset"}."don't reset") -> ()
                    n184 = Greater?(x=w852, y=9) -> (0:w858:bool)
                    n185 = Greater?(x=w853, y=29.0) -> (0:w857:bool)
                    n186 = And(x=w857, y=w858) -> (x .and. y?=w856:bool)
                    "c" <- w856
                    n187 = Select(t=T2."c", s=w856, f=T2."b") -> (s? t:f=w861:T2)
                    n188 = local write "part"(w861) -> ()
                    n189 = Multiply(x=0, y=w865) -> (x*y=w864:dbl)
                    "x distance currently being travelled" <- 3
                    "y distance currently being travelled" <- 1
                    "Step 2B" <- TRUE
                  }
                  frame "c" {
                    n190 = Multiply(x=0, y=w876) -> (x*y=w875:dbl)
                    n191 = for {
                      N: 1 -> [_]
                      n192 = local read "Pulses M1"() -> (w887:dbl)
                      n193 = local read "Pulses M2"() -> (w883:dbl)
                      n194 = local write "Has encoders been reset?"(enum16{"don't reset", "reset"}."reset") -> ()
                      n195 = Equal To 0?(x=w883) -> (x = 0?=w881:bool)
                      n196 = Equal To 0?(x=w887) -> (x = 0?=w882:bool)
                      n197 = And(x=w882, y=w881) -> (x .and. y?=w880:bool)
                      n198 = Select(t=T2."d", s=w880, f=T2."c") -> (s? t:f=w886:T2)
                      n199 = local write "part"(w886) -> ()
                    }
                    n200 = Multiply(x=0, y=w874) -> (x*y=w873:dbl)
                    "Step 2C" <- TRUE
                  }
                  frame "d" {
                    n201 = local write "Has encoders been reset?"(enum16{"don't reset", "reset"}."don't reset") -> ()
                    n202 = Multiply(x=1, y=w904) -> (x*y=w902:dbl)
                    n203 = Multiply(x="height", y=10) -> (x*y=w896:dbl)
                    n204 = local write "y distance currently being travelled"("height") -> ()
                    n205 = local write "x distance currently being travelled"(0) -> ()
                    n206 = Subtract(x=w896, y=1) -> (x-y=w893:dbl)
                    n207 = Multiply(x=-1, y=w901) -> (x*y=w900:dbl)
                    n208 = local read "calc distance y"() -> (w898:dbl)
                    n209 = Greater?(x=w898, y=w893) -> (0:w889:bool)
                    "Step 2D" <- w889
                    n210 = Select(t=T2."e", s=w889, f=T2."d") -> (s? t:f=w899:T2)
                    n211 = local write "part"(w899) -> ()
                  }
                  frame "e" {
                    n212 = Multiply(x=0, y=w911) -> (x*y=w910:dbl)
                    n213 = for {
                      N: 1 -> [_]
                      n214 = local read "Pulses M2"() -> (w915:dbl)
                      n215 = local read "Pulses M1"() -> (w916:dbl)
                      n216 = local write "Has encoders been reset?"(enum16{"don't reset", "reset"}."reset") -> ()
                      n217 = Equal To 0?(x=w915) -> (x = 0?=w921:bool)
                      n218 = Equal To 0?(x=w916) -> (x = 0?=w922:bool)
                      n219 = And(x=w922, y=w921) -> (x .and. y?=w920:bool)
                      n220 = Select(t=T2."f", s=w920, f=T2."e") -> (s? t:f=w914:T2)
                      n221 = local write "part"(w914) -> ()
                    }
                    n222 = Multiply(x=0, y=w907) -> (x*y=w908:dbl)
                  }
                  frame "f" {
                    n223 = Multiply(x=1.5, y=w928) -> (x*y=w927:dbl)
                    n224 = Multiply(x="length", y=10) -> (x*y=w935:dbl)
                    n225 = local read "calc distanc x"() -> (w938:dbl)
                    n226 = Subtract(x=w935, y=1) -> (x-y=w932:dbl)
                    n227 = local write "Has encoders been reset?"(enum16{"don't reset", "reset"}."don't reset") -> ()
                    n228 = local write "x distance currently being travelled"("length") -> ()
                    n229 = Greater?(x=w938, y=w932) -> (0:w923:bool)
                    "at 2f" <- w923
                    n230 = local write "y distance currently being travelled"(0) -> ()
                    n231 = Select(t=T2."g", s=w923, f=T2."f") -> (s? t:f=w937:T2)
                    n232 = Multiply(x=1.5, y=w925) -> (x*y=w924:dbl)
                    n233 = local write "part"(w937) -> ()
                  }
                  frame "g" {
                    n234 = Multiply(x=0, y=w944) -> (x*y=w945:dbl)
                    n235 = for {
                      N: 1 -> [_]
                      n236 = local read "Pulses M1"() -> (w949:dbl)
                      n237 = local read "Pulses M2"() -> (w948:dbl)
                      n238 = local write "Has encoders been reset?"(enum16{"don't reset", "reset"}."reset") -> ()
                      n239 = Equal To 0?(x=w948) -> (x = 0?=w955:bool)
                      n240 = Equal To 0?(x=w949) -> (x = 0?=w956:bool)
                      n241 = And(x=w956, y=w955) -> (x .and. y?=w954:bool)
                      n242 = Select(t=T2."h", s=w954, f=T2."g") -> (s? t:f=w951:T2)
                      n243 = local write "part"(w951) -> ()
                    }
                    n244 = Multiply(x=0, y=w941) -> (x*y=w942:dbl)
                  }
                  frame "h" {
                    n245 = local write "Has encoders been reset?"(enum16{"don't reset", "reset"}."don't reset") -> ()
                    n246 = Multiply(x=-1, y=w965) -> (x*y=w964:dbl)
                    n247 = local read "height"() -> (w962:dbl)
                    n248 = Multiply(x=w962, y=10) -> (x*y=w972:dbl)
                    n249 = local write "y distance currently being travelled"(w962) -> ()
                    n250 = Subtract(x=w972, y=1) -> (x-y=w969:dbl)
                    n251 = Multiply(x=1, y=w960) -> (x*y=w959:dbl)
                    n252 = local write "x distance currently being travelled"(0) -> ()
                    n253 = local read "calc distance y"() -> (w958:dbl)
                    n254 = Greater?(x=w958, y=w969) -> (0:w973:bool)
                    n255 = Select(t=T2."i", s=w973, f=T2."h") -> (s? t:f=w963:T2)
                    n256 = local write "part"(w963) -> ()
                    "Step 2H" <- TRUE
                  }
                  frame "i" {
                    n257 = Multiply(x=0, y=w979) -> (x*y=w980:dbl)
                    n258 = for {
                      N: 1 -> [_]
                      n259 = local read "Pulses M1"() -> (w985:dbl)
                      n260 = local read "Pulses M2"() -> (w984:dbl)
                      n261 = local write "Has encoders been reset?"(enum16{"don't reset", "reset"}."reset") -> ()
                      n262 = Equal To 0?(x=w984) -> (x = 0?=w990:bool)
                      n263 = Equal To 0?(x=w985) -> (x = 0?=w991:bool)
                      n264 = And(x=w991, y=w990) -> (x .and. y?=w989:bool)
                      n265 = Select(t=T2."j", s=w989, f=T2."i") -> (s? t:f=w983:T2)
                      n266 = local write "part"(w983) -> ()
                    }
                    n267 = Multiply(x=0, y=w976) -> (x*y=w977:dbl)
                  }
                  frame "j" {
                    (unwired) 1
                    n268 = Multiply(x=-1, y=w1002) -> (x*y=w1001:dbl)
                    n269 = local read "length"() -> (w995:dbl)
                    n270 = local read "calc distanc x"() -> (w997:dbl)
                    n271 = Multiply(x=w995, y=10) -> (x*y=w992:dbl)
                    n272 = local write "Has encoders been reset?"(enum16{"don't reset", "reset"}."don't reset") -> ()
                    n273 = local write "x distance currently being travelled"(w995) -> ()
                    n274 = Greater?(x=w997, y=w992) -> (0:w1006:bool)
                    n275 = local write "y distance currently being travelled"(0) -> ()
                    n276 = Select(t=T2."nothing", s=w1006, f=T2."j") -> (s? t:f=w996:T2)
                    n277 = Multiply(x=-1.08, y=w1000) -> (x*y=w999:dbl)
                    n278 = local write "part"(w996) -> ()
                    "Step 2J" <- TRUE
                  }
                  frame "nothing" {
                    n279 = Multiply(x=0, y=w1013) -> (x*y=w1012:dbl)
                    n280 = Multiply(x=0, y=w1011) -> (x*y=w1009:dbl)
                  }
                }
              }
              frame True {
                n281 = case shown="\"b\"" "part circle" {
                  frame "a" {
                    n282 = for {
                      N: 1 -> [_]
                      n283 = local read "Pulses M1"() -> (w1024:dbl)
                      n284 = local read "Pulses M2"() -> (w1023:dbl)
                      n285 = Equal To 0?(x=w1024) -> (x = 0?=w1026:bool)
                      n286 = Equal To 0?(x=w1023) -> (x = 0?=w1027:bool)
                      n287 = And(x=w1026, y=w1027) -> (x .and. y?=w1028:bool)
                      n288 = local write "Has encoders been reset?"(enum16{"don't reset", "reset"}."reset") -> ()
                      n289 = Select(t=T1."going down", s=w1028, f=T1."a") -> (s? t:f=w1021:T1)
                      n290 = local write "part circle"(w1021) -> ()
                      "circle reset" <- TRUE
                    }
                  }
                  frame "going down" {
                    n291 = local read "calc distance y"() -> (w1036:dbl)
                    n292 = Greater?(x=w1036, y=38) -> (0:w1032:bool)
                    n293 = local write "Has encoders been reset?"(enum16{"don't reset", "reset"}."don't reset") -> ()
                    n294 = Select(t=T1."going right", s=w1032, f=T1."going right") -> (s? t:f=w1031:T1)
                    n295 = local write "y distance currently being travelled"(-4) -> ()
                    n296 = local write "part circle"(w1031) -> ()
                    "down" <- TRUE
                  }
                  frame "going right" {
                    n297 = local write "Has encoders been reset?"(enum16{"don't reset", "reset"}."reset") -> ()
                    n298 = local write "part circle"(T1."b") -> ()
                    "right" <- TRUE
                  }
                  frame "b" {
                    n299 = local read "calc distanc x"() -> (w1054:dbl)
                    n300 = local read "Raduis"() -> (w1057:dbl)
                    n301 = local read "calc distance y"() -> (w1053:dbl)
                    n302 = Multiply(x=w1057, y=10) -> (x*y=w1056:dbl)
                    n303 = Subtract(x=w1056, y=1) -> (x-y=w1045:dbl)
                    n304 = local read "Raduis"() -> (w1048:dbl)
                    n305 = Multiply(x=-1, y=w1048) -> (x*y=w1047:dbl)
                    n306 = Greater?(x=w1054, y=w1045) -> (0:w1052:bool)
                    n307 = local write "y distance currently being travelled"(w1047) -> ()
                    n308 = Multiply(x=-1, y=w1045) -> (x*y=w1044:dbl)
                    n309 = Greater?(x=w1053, y=w1044) -> (0:w1051:bool)
                    n310 = local write "x distance currently being travelled"(w1048) -> ()
                    n311 = And(x=w1052, y=w1051) -> (x .and. y?=w1050:bool)
                    "b" <- w1050
                    n312 = local write "Has encoders been reset?"(enum16{"don't reset", "reset"}."don't reset") -> ()
                    n313 = Select(t=T1."c", s=w1050, f=T1."b") -> (s? t:f=w1041:T1)
                    n314 = local write "part circle"(w1041) -> ()
                  }
                  frame "c" {
                    n315 = for {
                      N: 1 -> [_]
                      n316 = local read "Pulses M1"() -> (w1067:dbl)
                      n317 = local read "Pulses M2"() -> (w1066:dbl)
                      n318 = Equal To 0?(x=w1067) -> (x = 0?=w1068:bool)
                      n319 = Equal To 0?(x=w1066) -> (x = 0?=w1069:bool)
                      n320 = local write "Has encoders been reset?"(enum16{"don't reset", "reset"}."reset") -> ()
                      n321 = And(x=w1068, y=w1069) -> (x .and. y?=w1063:bool)
                      "c" <- w1063
                      n322 = Select(t=T1."d", s=w1063, f=T1."c") -> (s? t:f=w1064:T1)
                      n323 = local write "part circle"(w1064) -> ()
                    }
                  }
                  frame "d" {
                    n324 = while {
                      i -> [w1079]
                      stop <- w1078 stop-if-true
                      n325 = for {
                        N: 50 -> [_]
                        tunnel: [w1082] -> w1072
                        i -> [w1087]
                        n326 = Increment(x=w1087) -> (x+1=w1083:i32)
                        "Numeric 2" <- w1083
                        n327 = Multiply(x=2, y=3.141592653589793) -> (x*y=w1084:dbl)
                        n328 = Divide(x=w1084, y=50) -> (x/y=w1086:dbl)
                        n329 = Multiply(x=w1086, y=w1083) -> (x*y=w1082:dbl)
                      }
                      n330 = Equal?(x=49, y=w1079) -> (x = y?=w1078:bool)
                      n331 = local write "Has encoders been reset?"(enum16{"don't reset", "reset"}."don't reset") -> ()
                      n332 = Cosine(x=w1072) -> (cos(x)=w1074:dbl)
                      n333 = Sine(x=w1072) -> (sin(x)=w1075:dbl)
                      n334 = Multiply(x=w1075, y="Raduis") -> (x*y=w1077:dbl)
                      n335 = Multiply(x=w1074, y="Raduis") -> (x*y=w1076:dbl)
                      n336 = local write "x distance currently being travelled"(w1076) -> ()
                      n337 = local write "y distance currently being travelled"(w1077) -> ()
                      "d" <- TRUE
                    }
                  }
                }
              }
            }
            "Numeric" <- 2
          }
        }
      }
    }
    "In drawing mode" <- w173
    n338 = Select(t=w172, s=w150, f=w170) -> (s? t:f=w169:dbl)
    n339 = Select(t=w171, s=w150, f=w168) -> (s? t:f=w167:dbl)
    n340 = And(x=w66, y=w59) -> (x .and. y?=w149:bool)
    n341 = Or(x=w210, y=w149) -> (x .or. y?=w209:bool)
    n342 = Or(x=w209, y="Motor stop") -> (x .or. y?=w211:bool)
    n343 = Or(x=w211, y="stop") -> (x .or. y?=w231:bool)
    n344 = Select(t=0.0, s=w231, f=w167) -> (s? t:f=w228:dbl)
    n345 = call-poly <vilib>:"DAQmx Write.vi"("task/channels in"=w237, "data"=w228, "error in"=w234) -> ("task out"=w238:refnum<k21>, "error out"=w239:errorcluster)  [unwired: 10 in, 1 out]
    n346 = Select(t=0.0 ("s? t:f"), s=w231, f=w169) -> (s? t:f=w229:dbl)
    n347 = call-poly <vilib>:"DAQmx Write.vi"("task/channels in"=w243, "data"=w229, "error in"=w233) -> ("task out"=w242:refnum<k21>, "error out"=w241:errorcluster)  [unwired: 10 in, 1 out]
    n348 = call <vilib>:"DAQmx Wait Until Done.vi"("task/channels in"=w242, "error in"=w241) -> ("error out"=w240:errorcluster)  [unwired: 12 in, 1 out]
    n349 = call <vilib>:"DAQmx Wait Until Done.vi"("task/channels in"=w238, "error in"=w239) -> ("error out"=w236:errorcluster)  [unwired: 12 in, 1 out]
    n350 = case shown="True" w126 {
      tunnel: w127 -> [w245 w246]
      frame False {
        n351 = call-poly <vilib>:"DAQmx Read.vi"("task/channels in"=w245) -> ("data"=w244:dbl)  [unwired: 12 in, 2 out]
        n352 = local write "Pulses M2"(w244) -> ()
      }
      frame True {
        n353 = local read "Has encoders been reset?"() -> (w247:enum16{"don't reset", "reset"})
        n354 = case shown="\"reset\"" w247 {
          tunnel: w246 -> [w249 w252]
          frame "don't reset", Default {
            n355 = call-poly <vilib>:"DAQmx Read.vi"("task/channels in"=w249) -> ("data"=→"Pulses M2":dbl)  [unwired: 12 in, 2 out]
          }
          frame "reset" {
            n356 = call <vilib>:"DAQmx Stop Task.vi"("task/channels in"=w252) -> ("task out"=w251:refnum<k21>)  [unwired: 13 in, 1 out]
            n357 = call <vilib>:"DAQmx Start Task.vi"("task/channels in"=w251) -> ("task out"=w253:refnum<k21>)  [unwired: 13 in, 1 out]
            n358 = call-poly <vilib>:"DAQmx Read.vi"("task/channels in"=w253) -> ("data"=w250:dbl)  [unwired: 12 in, 2 out]
            n359 = local write "Pulses M2"(w250) -> ()
          }
        }
      }
    }
    n360 = call "Number To Enum.vim"("number"=w163, "enum type"=enum16{"corner", "1st switch", "reverse"}."corner") -> ("number as enum"=→"Shape drawing steps":enum16{"corner", "1st switch", "reverse"})
    n361 = case shown="True" w126 {
      tunnel: w131 -> [w256 w261]
      tunnel: w130 -> [w257 w260]
      tunnel: [w254 w259] -> w129
      frame False {
        n362 = call-poly <vilib>:"DAQmx Read.vi"("task/channels in"=w256, "error in"=w257) -> ("data"=w255:dbl, "error out"=w254:errorcluster)  [unwired: 11 in, 1 out]
        n363 = local write "Pulses M1"(w255) -> ()
      }
      frame True {
        n364 = case shown="\"reset\"" "Has encoders been reset?" {
          tunnel: w261 -> [w265 w272]
          tunnel: w260 -> [w264 w271]
          tunnel: [w262 w273] -> w259
          frame "don't reset", Default {
            n365 = call-poly <vilib>:"DAQmx Read.vi"("task/channels in"=w265, "error in"=w264) -> ("data"=→"Pulses M1":dbl, "error out"=w262:errorcluster)  [unwired: 11 in, 1 out]
          }
          frame "reset" {
            n366 = call <vilib>:"DAQmx Stop Task.vi"("task/channels in"=w272, "error in"=w271) -> ("task out"=w270:refnum<k21>, "error out"=w269:errorcluster)  [unwired: 12 in]
            n367 = call <vilib>:"DAQmx Start Task.vi"("task/channels in"=w270, "error in"=w269) -> ("task out"=w268:refnum<k21>, "error out"=w267:errorcluster)  [unwired: 12 in]
            n368 = call-poly <vilib>:"DAQmx Read.vi"("task/channels in"=w268, "error in"=w267) -> ("data"=w266:dbl, "error out"=w273:errorcluster)  [unwired: 11 in, 1 out]
            n369 = local write "Pulses M1"(w266) -> ()
          }
        }
      }
    }
  }
  n370 = invoke on="motor 1" class="Slide (strict)" method="Reinit To Default"() -> ()  [unwired: 3 in, 3 out]
  n371 = call <vilib>:"Simple Error Handler.vi"("error source (\" \")"="you messed up" ("error source (\" \")"), "error in (no error)"=w48) -> ()  [unwired: 3 in, 5 out]
  n372 = call <vilib>:"Simple Error Handler.vi"("error source (\" \")"="you messed up" ("error source (\" \")"), "error in (no error)"=w45) -> ()  [unwired: 3 in, 5 out]
  n373 = call <vilib>:"DAQmx Clear Task.vi"("task in"=w27, "error in"=w25) -> ()  [unwired: 13 in, 1 out]
  n374 = call <vilib>:"DAQmx Clear Task.vi"("task in"=w17, "error in"=w14) -> ()  [unwired: 13 in, 1 out]
  n375 = call <vilib>:"DAQmx Clear Task.vi"("task in"=w18, "error in"=w15) -> ("error out"=w12:errorcluster)  [unwired: 13 in]
  n376 = call <vilib>:"DAQmx Clear Task.vi"("task in"=w16, "error in"=w13) -> ()  [unwired: 13 in, 1 out]
  n377 = call <vilib>:"Simple Error Handler.vi"("error in (no error)"=w12) -> ()  [unwired: 4 in, 5 out]
  n378 = call <vilib>:"Simple Error Handler.vi"("error source (\" \")"="you messed up" ("error source (\" \")"), "error in (no error)"=w10) -> ()  [unwired: 3 in, 5 out]
